vi "normalisation.vi"(11 "intensity matrix":dbl[][](array[numeric])) -> (3 "Array":dbl[][](array[numeric]))   [LabVIEW 2015]
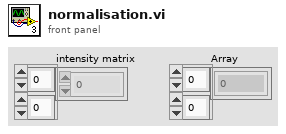
[diagram p1: front panel]
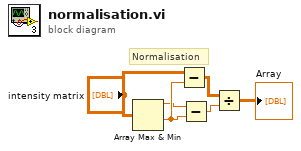
[diagram p0: block diagram]
diagram:
  # "Normalisation"
  n1 = Array Max & Min(array="intensity matrix") -> (max value=w1:dbl, min value=w2:dbl)  [unwired: 2 out]
  n2 = Subtract(x="intensity matrix", y=w2) -> (x-y=w4:dbl[][])
  n3 = Subtract(x=w1, y=w2) -> (x-y=w3:dbl)
  n4 = Divide(x=w4, y=w3) -> (x/y=→"Array":dbl[][])
